vi "LCR_OpenShortCompensation.vi"(6 "Freq":dbl=29568.503937007874, 7 "UseCorrection":bool=TRUE, 9 "Cal Cluster":T1={"ESL_Cal"=2e-07, "ESR_Cal"=0.001, "Cp_Cal"=0.0, "Rp_Cal"=0.0, "RLoad"=1000000000.0, "RLoad_Meas"=1000000000.0} {"RLoad_Meas" format="%#_6p"; "RLoad" format="%#_6p"}, 10 "Phase Z Meas Deg":dbl=-274.14043501202957, 11 "Mag Z Meas":dbl=0.05495335386432602) -> (0 "Z DUT":cdb=0.002970463906317392-185.81585831552346i, 2 "Phase Z DUT":dbl=-89.99908406609342, 3 "Mag Z DUT":dbl=185.81585833926647)   [LabVIEW 2021]
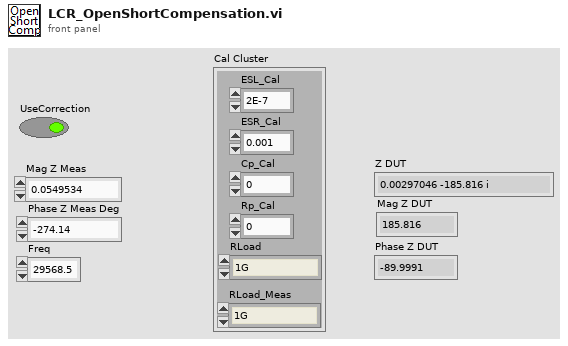
[diagram p1: front panel]
types:
  T1 = cluster{"ESL_Cal":dbl, "ESR_Cal":dbl, "Cp_Cal":dbl, "Rp_Cal":dbl, "RLoad":dbl, "RLoad_Meas":dbl}
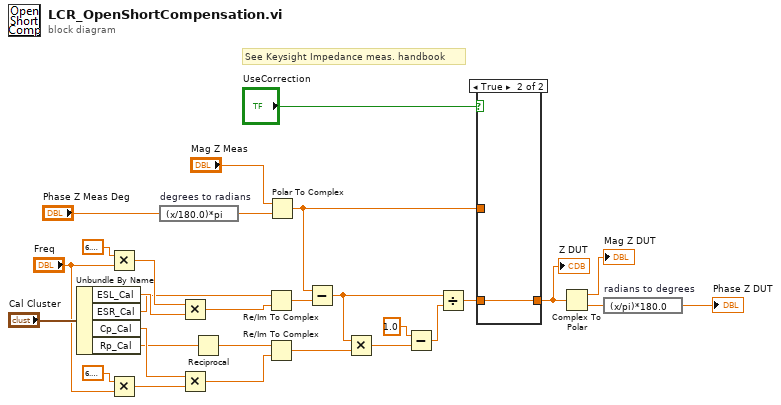
[diagram p0: block diagram]
diagram:
  # "See Keysight Impedance meas. handbook"
  n1 = Unbundle By Name("Cal Cluster") -> ("ESL_Cal"=w10:dbl, "ESR_Cal"=w9:dbl, "Cp_Cal"=w6:dbl, "Rp_Cal"=w4:dbl)
  n2 = Multiply(x=6.283185307179586, y="Freq") -> (x*y=w14:dbl)
  n3 = Multiply(x=6.283185307179586, y="Freq") -> (x*y=w7:dbl)
  n4 = expression code="(x/180.0)*pi" "degrees to radians"("Phase Z Meas Deg") -> (w22:dbl)
  n5 = Multiply(x=w14, y=w10) -> (x*y=w13:dbl)
  n6 = Multiply(x=w6, y=w7) -> (x*y=w5:dbl)
  n7 = Reciprocal(x=w4) -> (1/x=w3:dbl)
  n8 = Re/Im To Complex(1:w13, 2:w9) -> (0:w12:cdb)
  n9 = Re/Im To Complex(1:w5, 2:w3) -> (0:w1:cdb)
  n10 = Polar To Complex(1:w22, 2:"Mag Z Meas") -> (0:w18:cdb)
  n11 = Subtract(x=w18, y=w12) -> (x-y=w25:cdb)
  n12 = Multiply(x=w25, y=w1) -> (x*y=w27:cdb)
  n13 = Subtract(x=1.0, y=w27) -> (x-y=w26:cdb)
  n14 = Divide(x=w25, y=w26) -> (x/y=w20:cdb)
  n15 = case shown="True" "UseCorrection" {
    tunnel: w20 -> [_ w31]
    tunnel: [w30 w31] -> w19
    tunnel: w18 -> [w30 _]
    frame False {
    }
    frame True {
    }
  }
  "Z DUT" <- w19
  n16 = Complex To Polar(r * e^(i*theta)=w19) -> (r=→"Mag Z DUT":dbl, theta=w17:dbl)
  n17 = expression code="(x/pi)*180.0" "radians to degrees"(w17) -> (→"Phase Z DUT":dbl)
